vi "oa_Extract Even Angle Signal at Revolution Index (1 Channel).vi"(8 "index in range":bool, 9 "block size":i32=1024 min=2, 10 "rev index":dbl, 11 "even angle signal":cluster{"r0":dbl, "dr":dbl, "Y":dbl[]}={"r0"=0.0, "dr"=1.0, "Y"=[]} {"r0" format="%.2p"; "dr" format="%.2p"; "Y" format="%.2f"}) -> (2 "even angle signal for buffer":cluster{"r0":dbl, "dr":dbl, "Y":dbl[]}={"r0"=0.0, "dr"=1.0, "Y"=[]} {"r0" format="%.2p"; "dr" format="%.2p"; "Y" format="%.2f"}, 3 "even angle signal out":cluster{"r0":dbl, "dr":dbl, "Y":dbl[]}={"r0"=0.0, "dr"=1.0, "Y"=[]} {"r0" format="%.2p"; "dr" format="%.2p"; "Y" format="%.2f"})   [LabVIEW 2017, in "SoundVib_OAUtility.lvlib"]
uses:
  <vilib>/addons/Sound and Vibration/Order Analysis/Utility/SoundVib_OAUtility.lvlib
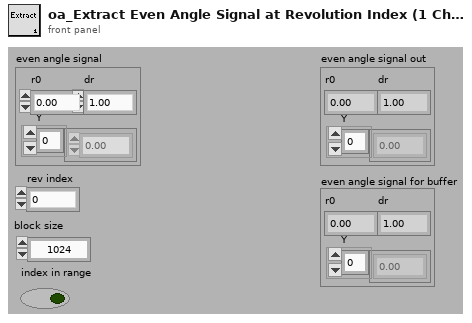
[diagram p1: front panel]
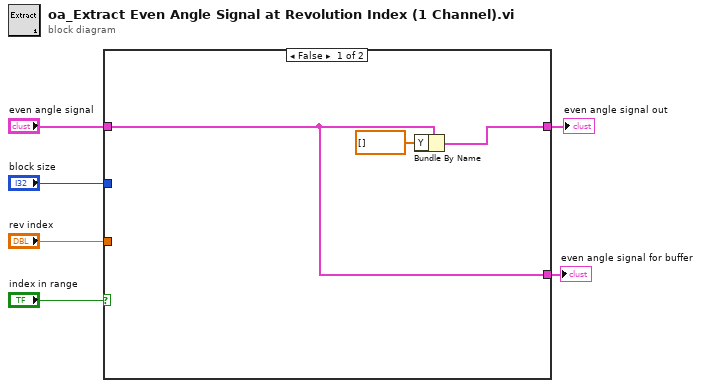
[diagram p0: block diagram]
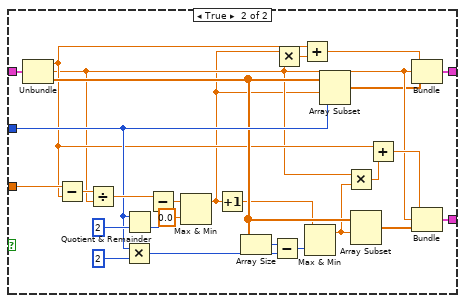
[diagram p2: hidden frame]
diagram:
  n1 = case shown="False" "index in range" {
    tunnel: "even angle signal" -> [w9 w36]
    tunnel: [w9 w29] -> w4
    tunnel: [w7 w31] -> w3
    tunnel: "rev index" -> [_ w35]
    tunnel: "block size" -> [_ w27]
    frame False {
      n2 = Bundle By Name(cluster=w9, "Y"=dbl[] []) -> (w7:cluster{"r0":dbl, "dr":dbl, "Y":dbl[]})
    }
    frame True {
      n3 = Unbundle(w36) -> ("r0"=w18:dbl, "dr"=w14:dbl, "Y"=w25:dbl[])
      n4 = Subtract(x=w35, y=w18) -> (x-y=w34:dbl)
      n5 = Divide(x=w34, y=w14) -> (x/y=w28:dbl)
      n6 = Multiply(x=w27, y=2) -> (x*y=w23:i32)
      n7 = Quotient & Remainder(x=w27, y=2) -> (floor(x/y)=w32:i32)  [unwired: 1 out]
      n8 = Subtract(x=w28, y=w32) -> (x-y=w13:dbl)
      n9 = Max & Min(x=w13, y=0.0) -> (max(x,y)=w11:dbl)  [unwired: 1 out]
      n10 = Increment(x=w11) -> (x+1=w21:dbl)
      n11 = Array Size(array=w25) -> (size(s)=w24:i32)
      n12 = Subtract(x=w24, y=w23) -> (x-y=w22:i32)
      n13 = Multiply(x=w11, y=w14) -> (x*y=w19:dbl)
      n14 = Add(x=w18, y=w19) -> (x+y=w17:dbl)
      n15 = Max & Min(x=w21, y=w22) -> (max(x,y)=w16:dbl)  [unwired: 1 out]
      n16 = Array Subset(array=w25, index=w11, length=w27) -> (w10:dbl[])
      n17 = Multiply(x=w14, y=w16) -> (x*y=w15:dbl)
      n18 = Array Subset(array=w25, index=w16) -> (w30:dbl[])  [unwired: 1 in]
      n19 = Add(x=w18, y=w15) -> (x+y=w20:dbl)
      n20 = Bundle(w17, "dr"=w14, w10) -> (w31:cluster{dbl, "dr":dbl, dbl[]})  [unwired: 1 in]
      n21 = Bundle(w20, "dr"=w14, w30) -> (w29:cluster{dbl, "dr":dbl, dbl[]})  [unwired: 1 in]
    }
  }
  "even angle signal for buffer" <- w4
  "even angle signal out" <- w3
